vi "PRUEBA_A_IO.vi"() -> ()   [LabVIEW 2025]
panel:
  out "Slide":u8(slide) scale=0.0..255.0
  in  "Pin":u8=25 min=25 max=26
  out "Voltaje":dbl
  in  "stop":bool
  in  "VISA resource name":refnum<visa-resource-name>
  out "error out":errorcluster
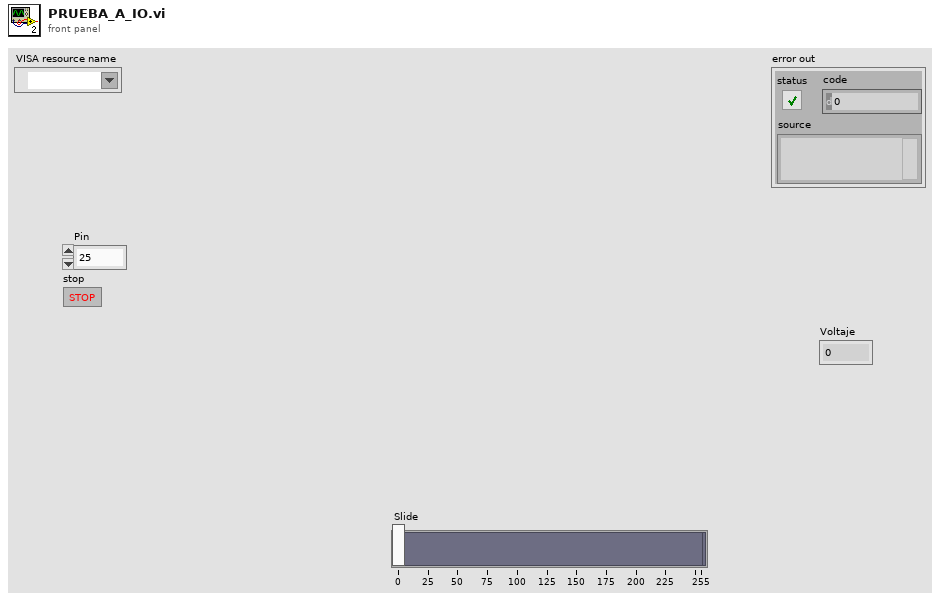
[diagram p1: front panel]
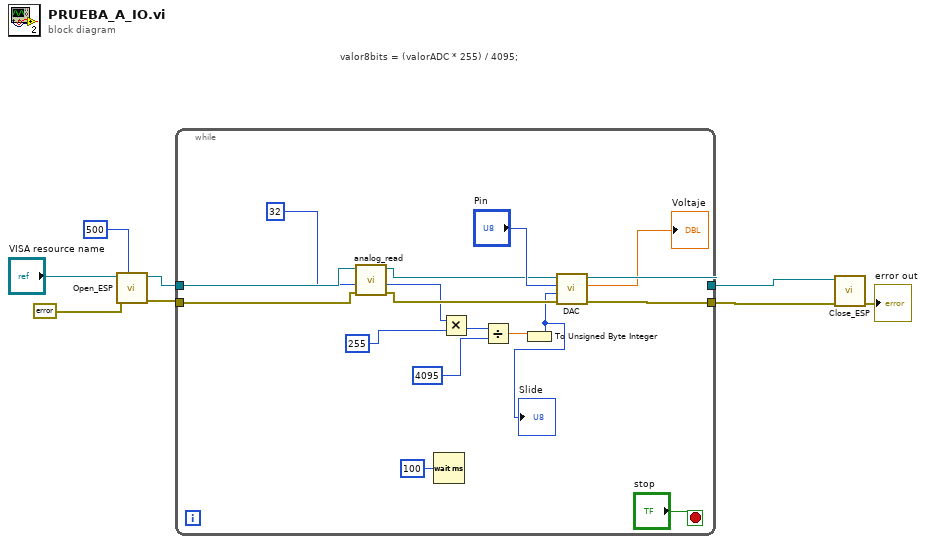
[diagram p0: block diagram]
diagram:
  # "valor8bits = (valorADC * 255) / 4095;"
  n1 = call "Open_ESP.vi"("timeout (10sec)"=u32 500, "error in (no error)"=errorcluster {"status"=FALSE, "code"=0, "source"=""}, "VISA resource name"="VISA resource name") -> ("error out"=w7:errorcluster, "VISA resource name out"=w8:refnum<visa-resource-name>)  [unwired: 7 in]
  n2 = while {
    tunnel: w8 -> [w17]
    tunnel: [w25] -> w6
    tunnel: w7 -> [w18]
    tunnel: [w24] -> w5
    stop <- "stop" stop-if-true
    n3 = call "analog_read.vi"("error in (no error)"=w18, "Pin"=u8 32, "VISA resource name"=w17) -> ("error out"=w19:errorcluster, "Analog read"=w15:u16, "VISA resource name out"=w20:refnum<visa-resource-name>)  [unwired: 6 in]
    n4 = Wait (ms)(milliseconds to wait=u32 100) -> ()  [unwired: 1 out]
    n5 = Multiply(x=w15, y=255) -> (x*y=w13:i32)
    n6 = Divide(x=w13, y=4095) -> (x/y=w11:dbl)
    n7 = To Unsigned Byte Integer(number=w11) -> (unsigned 8bit integer=w10:u8)
    "Slide" <- w10
    n8 = call "DAC.vi"("error in (no error)"=w19, "DAC"=w10, "Pin"="Pin", "VISA resource name"=w20) -> ("error out"=w24:errorcluster, "Voltaje"=→"Voltaje":dbl, "VISA resource name out"=w25:refnum<visa-resource-name>)  [unwired: 5 in]
  }
  n9 = call "Close_ESP.vi"("error in (no error)"=w5, "VISA resource name"=w6) -> ("error out"=→"error out":errorcluster)  [unwired: 9 in]
